vi "Do.vi"(8 "error in (no error)":errorcluster, 10 "Actor in":refnum<class "Actor.lvclass">, 11 "Create Channel Arbitrary Waveform I32 [ACH] Msg":refnum<class "Create Channel Arbitrary Waveform I32 [ACH] Msg.lvclass">) -> (0 "error out":errorcluster, 2 "Actor out":refnum<class "Actor.lvclass">)   [LabVIEW 2014, in "CS++Fgen.lvlib" / "Create Channel Arbitrary Waveform I32 [ACH] Msg.lvclass"]
doc: "This VI delivers the message to the actor by calling the appropriate method(s) on the actor."
uses:
  Create Channel Arbitrary Waveform I32 [ACH] Msg.lvclass
  <vilib>/ActorFramework/Actor/Actor.lvclass
  CS++Fgen/CS++Fgen.lvclass
  CSPP_Core/Actors/CS++PVMonitor Messages/CS++PVUpdate Msg/CS++PVUpdate Msg.lvclass/CS++PVUpdate Msg.ctl
  CSPP_Core/Classes/CS++ProcessVariables/ProcessVariable/PV.lvclass/PV.ctl
  Create Channel Arbitrary Waveform I32 [ACH] Msg.lvclass/Create Channel Arbitrary Waveform I32 [ACH] Msg.ctl
  CSPP_Core/Classes/CS++ProcessVariables/ProcessVariable/PV.lvclass
  CSPP_Core/Actors/CS++PVMonitor Messages/CS++PVUpdate Msg/CS++PVUpdate Msg.lvclass
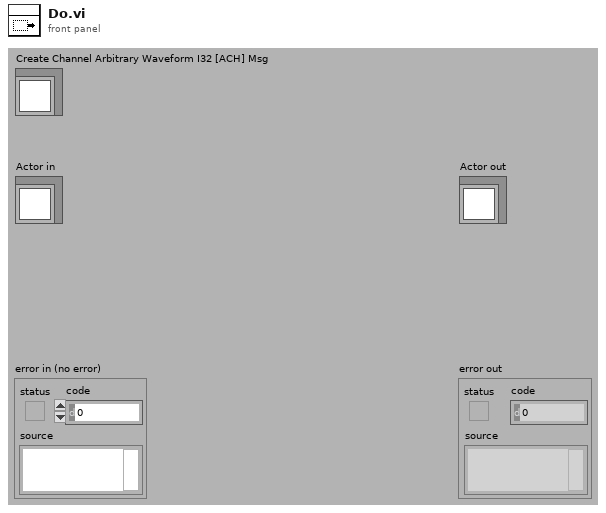
[diagram p1: front panel]
types:
  T1 = cluster{"Waveform Data Array":i32[], "Channel Name (\"\")":string}
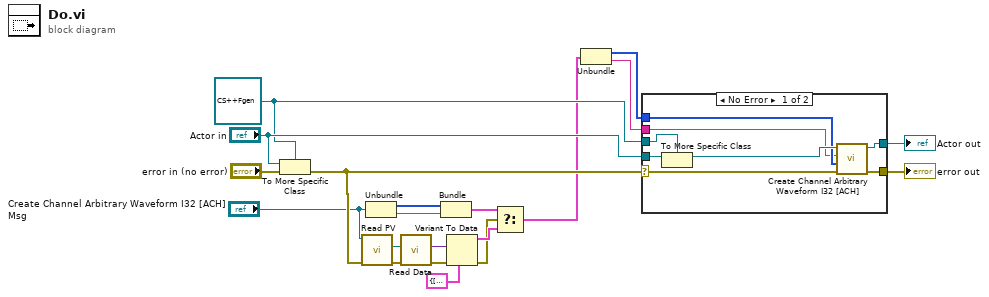
[diagram p0: block diagram]
diagram:
  w16 = refnum<class "CS++Fgen.lvclass"> refnum ("Actor in")
  n1 = To More Specific Class(target class=w16, reference="Actor in", error in="error in (no error)") -> (error out=w4:errorcluster)  [unwired: 1 out]
  n2 = call "Read PV.vi"("error in (no error)"=w4, "CS++PVUpdate Msg in"="Create Channel Arbitrary Waveform I32 [ACH] Msg") -> ("error out"=w7:errorcluster, "PV"=w13:refnum<class "PV.lvclass">)  [unwired: 7 in, 1 out]
  n3 = Unbundle("Create Channel Arbitrary Waveform I32 [ACH] Msg") -> (w8:i32[], w10:string)
  n4 = call "Read Data.vi"("error in (no error)"=w7, "PV in"=w13) -> ("error out"=w6:errorcluster, "Data"=w11:variant)  [unwired: 7 in, 1 out]
  n5 = Bundle("Waveform Data Array"=w8, "Channel Name (\"\")"=w10) -> (w9:T1)  [unwired: 1 in]
  n6 = Variant To Data(error in=w6, type=T1 {"Waveform Data Array"=[], "Channel Name (\"\")"="CHANNEL1"} ("Cluster of class private data"), Variant=w11) -> (data=w12:T1, error out=w5:errorcluster)
  n7 = Select(t=w9, s=w5, f=w12) -> (s? t:f=w2:T1)
  n8 = Unbundle(w2) -> ("Waveform Data Array"=w15:i32[], "Channel Name (\"\")"=w14:string)
  n9 = case shown="No Error" w4 {
    selector: w4 -> [w26 w30]
    tunnel: [w28 w30] -> w19
    tunnel: [w27 w29] -> w18
    tunnel: "Actor in" -> [w25 w29]
    tunnel: w16 -> [w24 _]
    tunnel: w15 -> [w22 _]
    tunnel: w14 -> [w21 _]
    frame No Error {
      n10 = To More Specific Class(target class=w24, reference=w25) -> (specific class reference=w23:refnum<class "CS++Fgen.lvclass">)  [unwired: 1 in, 1 out]
      n11 = call "Create Channel Arbitrary Waveform I32 [ACH].vi"("error in (no error)"=w26, "Waveform Data Array"=w22, "Channel Name (\"\")"=w21, "CS++Fgen in"=w23) -> ("error out"=w28:errorcluster, "CS++Fgen out"=w27:refnum<class "CS++Fgen.lvclass">)  [unwired: 5 in, 1 out]
    }
    frame Error {
      # "If type check fails, pass the original object out again."
    }
  }
  "error out" <- w19
  "Actor out" <- w18
